vi "AB_Engine_WriteVersionInfoMac.vi"(6 "set CFBundleIdentifier":bool, 8 "error in (no error)":errorcluster, 9 "version info":T1 {"FileType" items=["VFT_UNKNOWN", "VFT_APP", "VFT_DLL", "VFT_DRV", "VFT_FONT", "VFT_VXD", "-", "VFT_STATIC_LIB"]}, 11 "FilePath":path) -> (0 "error out":errorcluster)   [LabVIEW 2020]
uses:
  <vilib>/AppBuilder/AB_Version_Info.ctl
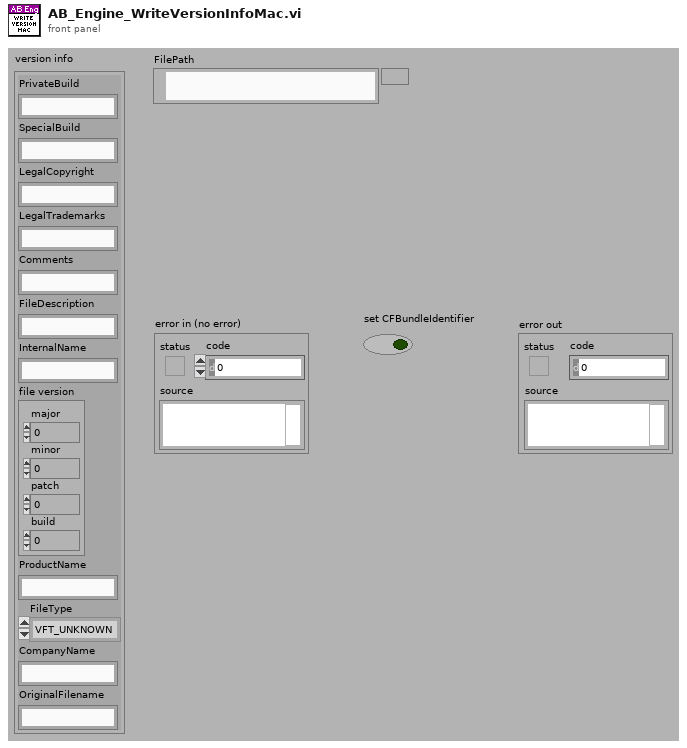
[diagram p1: front panel]
types:
  T1 = typedef "AB_Version_Info.ctl" = cluster{"PrivateBuild":string, "SpecialBuild":string, "LegalCopyright":string, "LegalTrademarks":string, "Comments":string, "FileDescription":string, "InternalName":string, "file version":cluster{"major":u16, "minor":u16, "patch":u16, "build":u16}, "ProductName":string, "FileType":u16, "CompanyName":string, "OriginalFilename":string}
  T2 = enum16{"open", "replace", "create", "open or create", "replace or create", "replace or create with confirmation"}
  T3 = cluster{"major":u16, "minor":u16, "patch":u16, "build":u16}
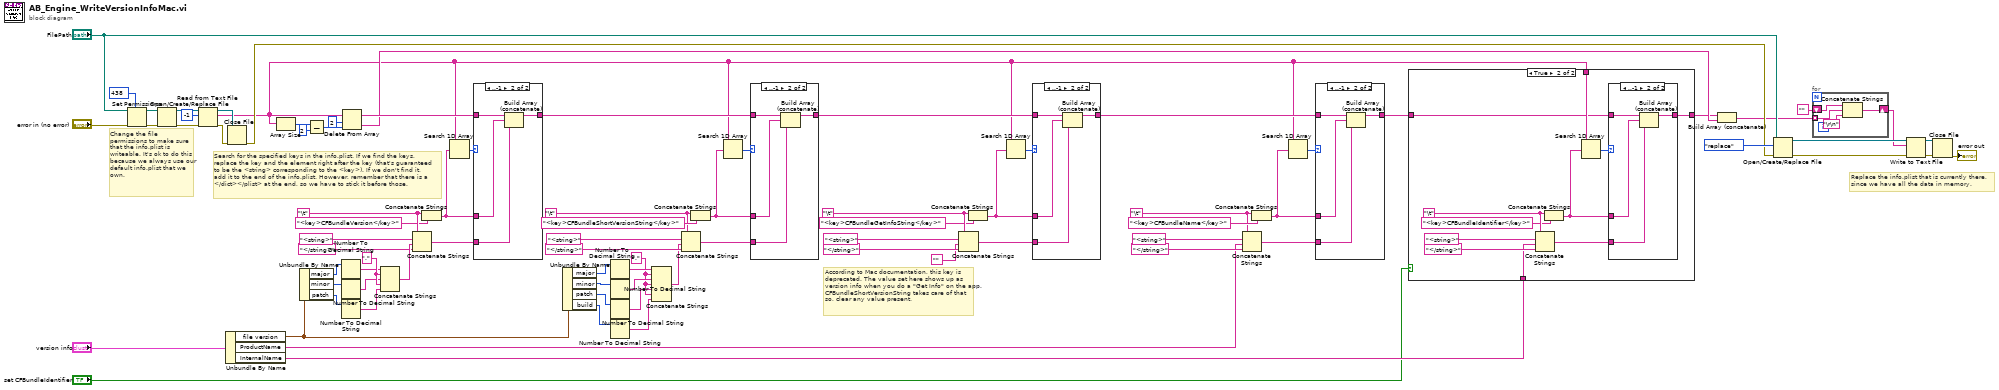
[diagram p0: block diagram]
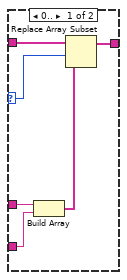
[diagram p3: hidden frame]
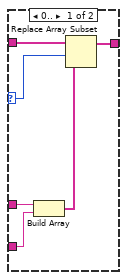
[diagram p4: hidden frame]
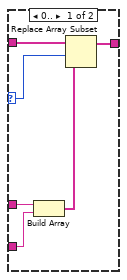
[diagram p5: hidden frame]
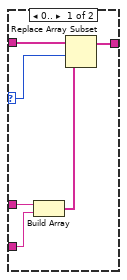
[diagram p6: hidden frame]
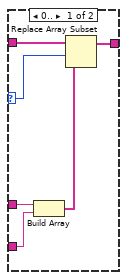
[diagram p7: hidden frame]
diagram:
  w31 = "\t"
  w40 = "\t"
  w48 = "."
  w60 = "\t"
  w76 = "."
  w70 = "\t"
  # "According to Mac documentation, this key is deprecated. The value set here shows up as version info when you do a \"Get Info\" on the app. CFBundleShortVersionString takes care of that so, clear any value present."
  # "Change the file permissions to make sure that the info.plist is writeable. It's ok to do this because we always use our default info.plist that we own."
  # "Replace the info.plist that is currently there,\nsince we have all the data in memory."
  # "Search for the specified keys in the info.plist. If we find the keys,\nreplace the key and the element right after the key (that's guaranteed\nto be the <string> corresponding to the <key>). If we don't find it,\nadd it to the end of the info.plist. However, remember that there is a\n</dict></plist> at the end, so we have to stick it before those."
  n1 = Set Permissions(7:i16 438 ("permissions"), 8:"error in (no error)", 11:"FilePath") -> (0:w12:errorcluster, 3:w14:path)  [unwired: 2 in]
  n2 = Open/Create/Replace File(file path (use dialog)=w14, error in=w12) -> (refnum out=w84:refnum<file>, error out=w28:errorcluster)  [unwired: 4 in, 1 out]
  n3 = Read from Text File(file (use dialog)=w84, count=-1, error in=w28) -> (refnum out=w29:refnum<file>, text=w8:string[], error out=w27:errorcluster)  [unwired: 1 in, 1 out]
  n4 = Unbundle By Name("version info") -> ("file version"=w50:T3, "ProductName"=w30:string, "InternalName"=w5:string)
  n5 = Close File(refnum=w29, error in=w27) -> (error out=w21:errorcluster)  [unwired: 1 out]
  n6 = Array Size(array=w8) -> (size(s)=w68:i32)
  n7 = Unbundle By Name(w50) -> ("major"=w73:u16, "minor"=w72:u16, "patch"=w71:u16)
  n8 = Subtract(x=w68, y=2) -> (x-y=w66:i32)
  n9 = Number To Decimal String(number=w73) -> (decimal integer string=w74:string)  [unwired: 1 in]
  n10 = Number To Decimal String(number=w72) -> (decimal integer string=w75:string)  [unwired: 1 in]
  n11 = Number To Decimal String(number=w71) -> (decimal integer string=w77:string)  [unwired: 1 in]
  n12 = Delete From Array(array=w8, length=2, index=w66) -> (deleted portion=w10:string[], array with subset deleted=w64:string[])
  n13 = Concatenate Strings(w74, w76, w75, w76, w77) -> (w80:string)
  n14 = Concatenate Strings(w70, "<string>", w80, "</string>") -> (w63:string)
  n15 = Concatenate Strings(w70, "<key>CFBundleVersion</key>") -> (w19:string)
  n16 = Search 1D Array(1D array=w8, element=w19) -> (index of element=w81:i32)  [unwired: 1 in]
  n17 = case shown="..-1" w81 {
    selector: w81 -> [w89 _]
    tunnel: w64 -> [w90 w94]
    tunnel: w19 -> [w88 w93]
    tunnel: w63 -> [w87 w92]
    tunnel: [w85 w91] -> w45
    frame 0.. {
      n18 = Build Array(w88, w87) -> (w86:string[])
      n19 = Replace Array Subset(array=w90, new element=w86, index=w89) -> (w85:string[])
    }
    frame ..-1 {
      n20 = Build Array (concatenate)(w94, w93, w92) -> (w91:string[])
    }
  }
  n21 = Unbundle By Name(w50) -> ("major"=w57:u16, "minor"=w58:u16, "patch"=w59:u16, "build"=w49:u16)
  n22 = Number To Decimal String(number=w57) -> (decimal integer string=w56:string)  [unwired: 1 in]
  n23 = Number To Decimal String(number=w58) -> (decimal integer string=w55:string)  [unwired: 1 in]
  n24 = Number To Decimal String(number=w59) -> (decimal integer string=w54:string)  [unwired: 1 in]
  n25 = Number To Decimal String(number=w49) -> (decimal integer string=w47:string)  [unwired: 1 in]
  n26 = Concatenate Strings(w56, w48, w55, w48, w54, w48, w47) -> (w51:string)
  n27 = Concatenate Strings(w60, "<string>", w51, "</string>") -> (w46:string)
  n28 = Concatenate Strings(w60, "<key>CFBundleShortVersionString</key>") -> (w18:string)
  n29 = Search 1D Array(1D array=w8, element=w18) -> (index of element=w62:i32)  [unwired: 1 in]
  n30 = case shown="..-1" w62 {
    selector: w62 -> [w99 _]
    tunnel: w45 -> [w100 w104]
    tunnel: w18 -> [w98 w103]
    tunnel: w46 -> [w97 w102]
    tunnel: [w95 w101] -> w44
    frame 0.. {
      n31 = Build Array(w98, w97) -> (w96:string[])
      n32 = Replace Array Subset(array=w100, new element=w96, index=w99) -> (w95:string[])
    }
    frame ..-1 {
      n33 = Build Array (concatenate)(w104, w103, w102) -> (w101:string[])
    }
  }
  n34 = Concatenate Strings(w40, "<string>", "", "</string>") -> (w38:string)
  n35 = Concatenate Strings(w40, "<key>CFBundleGetInfoString</key>") -> (w17:string)
  n36 = Search 1D Array(1D array=w8, element=w17) -> (index of element=w43:i32)  [unwired: 1 in]
  n37 = case shown="..-1" w43 {
    selector: w43 -> [w109 _]
    tunnel: w44 -> [w110 w114]
    tunnel: w17 -> [w108 w113]
    tunnel: w38 -> [w107 w112]
    tunnel: [w105 w111] -> w32
    frame 0.. {
      n38 = Build Array(w108, w107) -> (w106:string[])
      n39 = Replace Array Subset(array=w110, new element=w106, index=w109) -> (w105:string[])
    }
    frame ..-1 {
      n40 = Build Array (concatenate)(w114, w113, w112) -> (w111:string[])
    }
  }
  n41 = Concatenate Strings(w31, "<string>", w30, "</string>") -> (w37:string)
  n42 = Concatenate Strings(w31, "<key>CFBundleName</key>") -> (w16:string)
  n43 = Search 1D Array(1D array=w8, element=w16) -> (index of element=w33:i32)  [unwired: 1 in]
  n44 = case shown="..-1" w33 {
    selector: w33 -> [w119 _]
    tunnel: w32 -> [w120 w124]
    tunnel: w16 -> [w118 w123]
    tunnel: w37 -> [w117 w122]
    tunnel: [w115 w121] -> w7
    frame 0.. {
      n45 = Build Array(w118, w117) -> (w116:string[])
      n46 = Replace Array Subset(array=w120, new element=w116, index=w119) -> (w115:string[])
    }
    frame ..-1 {
      n47 = Build Array (concatenate)(w124, w123, w122) -> (w121:string[])
    }
  }
  n48 = case shown="True" "set CFBundleIdentifier" {
    tunnel: w8 -> [_ w129]
    tunnel: w7 -> [w125 w128]
    tunnel: [w125 w127] -> w6
    tunnel: w5 -> [_ w126]
    frame False {
    }
    frame True {
      w135 = "\t"
      n49 = Concatenate Strings(w135, "<string>", w126, "</string>") -> (w130:string)
      n50 = Concatenate Strings(w135, "<key>CFBundleIdentifier</key>") -> (w136:string)
      n51 = Search 1D Array(1D array=w129, element=w136) -> (index of element=w134:i32)  [unwired: 1 in]
      n52 = case shown="..-1" w134 {
        selector: w134 -> [w141 _]
        tunnel: w128 -> [w142 w146]
        tunnel: w136 -> [w140 w145]
        tunnel: w130 -> [w139 w144]
        tunnel: [w137 w143] -> w127
        frame 0.. {
          n53 = Build Array(w140, w139) -> (w138:string[])
          n54 = Replace Array Subset(array=w142, new element=w138, index=w141) -> (w137:string[])
        }
        frame ..-1 {
          n55 = Build Array (concatenate)(w146, w145, w144) -> (w143:string[])
        }
      }
    }
  }
  n56 = Build Array (concatenate)(w6, w10) -> (w2:string[])
  n57 = Open/Create/Replace File(file path (use dialog)="FilePath", error in=w21, operation (0:open)=T2."replace") -> (refnum out=w25:refnum<file>, error out=w24:errorcluster)  [unwired: 3 in, 1 out]
  n58 = for {
    shift-right: [w150] -> w1
    shift-left: "" -> [w149]
    tunnel: w2 -> [w148] mode=indexing
    n59 = Concatenate Strings(w149, w148, "\r\n") -> (w150:string)
  }
  n60 = Write to Text File(file (use dialog)=w25, text=w1, error in=w24) -> (refnum out=w23:refnum<file>, error out=w22:errorcluster)  [unwired: 1 in, 1 out]
  n61 = Close File(refnum=w23, error in=w22) -> (error out=→"error out":errorcluster)  [unwired: 1 out]
